vi "SDI-12 Multiple Operations.vi"() -> ()   [LabVIEW 2015]
doc: "A general set of examples of the SDI-12 API for a generic sensor. A tab control separates each example, and contains the following examples:\n1. Read Single.\n2. Read Multiple.\n3. Acknowledge Active.\n4. Change Address.\n5. Address Query.\n6. Send Identification."
uses:
  SDI-12.lvlib
panel:
  in  "Example Mode":T1(tab)=enum."Read Multiple"
  out "Address Out":string="a" caption="sensor address out"
  out "Number of Measurements Out":i32
  out "Measurements Out":dbl[](array[numeric])
  in  "Measurement Type In (Normal)":i32(ring) items=["Normal", "Concurrent", "Continuous"]
  out "Parameter Out":i32(ring) items=["0", "1", "2", "3", "4", "5", "6", "7", "8", "9"]
  in  "Parameter In (0)":i32(ring) items=["0", "1", "2", "3", "4", "5", "6", "7", "8", "9"]
  in  "CRC (False)":bool
  out "CRC Out":bool
  out "Measurement Type Out":i32(ring) items=["Normal", "Concurrent", "Continuous"]
  out "Time (s)":dbl
  out "Read Multiple: Error Array Out":errorcluster[](array[cluster])
  out "Number of Measurements Out Array":i32[](array[numeric])
  out "Measurements Out":dbl[][](array[numeric])
  in  "Measurement Type In (Normal)":i32(ring) items=["Normal", "Concurrent", "Continuous"]
  in  "Sensor Address In Array":string[](array[string])=["b", "b", "b"]
  in  "Parameter In Array (0)":i32[](array[ring])=[0, 0, 0] items=["0", "1", "2", "3", "4", "5", "6", "7", "8", "9"]
  in  "CRC In Array (False)":bool[](array[boolean])=[TRUE, FALSE, TRUE]
  out "Sensor Active?":bool
  out "Address Changed Successfully?":bool
  in  "New Address In":string="b"
  out "Query Address Returned":string
  out "Query Response?":bool
  out "Identification: Address":string
  out "SDI-12 Compatibility Number":dbl
  out "Company Name":string
  out "Sensor Model Number":string
  out "Sensor Version":string
  out "Serial Number":string
  in  "Error In (No Error)":errorcluster
  in  "Sensor Address In":string="0"
  in  "RS232 Port In":refnum<visa-resource-name>="COM11"
  out "Error Out":errorcluster
  # "Instructions:\n1.  Select the RS232 port that is connected to the SDI-12.\n2.  Enter a sensor address (not used for Read Multiple).\n3.  Select the desired test from the Example Mode Tab Control."
  # "4.  Select a Measurement type, a Parameter value,\n     and enable or disable CRC.\n5.  Run this VI."
  # "deg C"
  # "pH"
  # "specific conductance"
  # "salinity or TDS"
  # "DO % saturation"
  # "DO mg/L"
  # "ORP"
  # "depth"
  # "battery"
  # "4.  Enter an array of addresses of the sensors to measure.  All input arrays should be the same size.  The combined settings of each array at a single index value correspond to the settings of a single measurement. \n5.  Select a Measurement Type for all sensors.\n6.  Select an array of CRC settings.\n7.  Select an array of Parameter values if your sensor(s) support additional measurements by parameter value.  For example, for a single sensor parameter 0 (default) could be temperature, and parameter 1 could be humidity.\n8.  Run this VI."
  # "deg C"
  # "pH"
  # "specific conductance"
  # "salinity or TDS"
  # "DO % saturation"
  # "DO mg/L"
  # "ORP"
  # "depth"
  # "battery"
  # "4.  Run this VI."
  # "4.  Select the desired new address.\n5.  Run this VI."
  # "4.  Run this VI."
  # "4.  Run this VI."
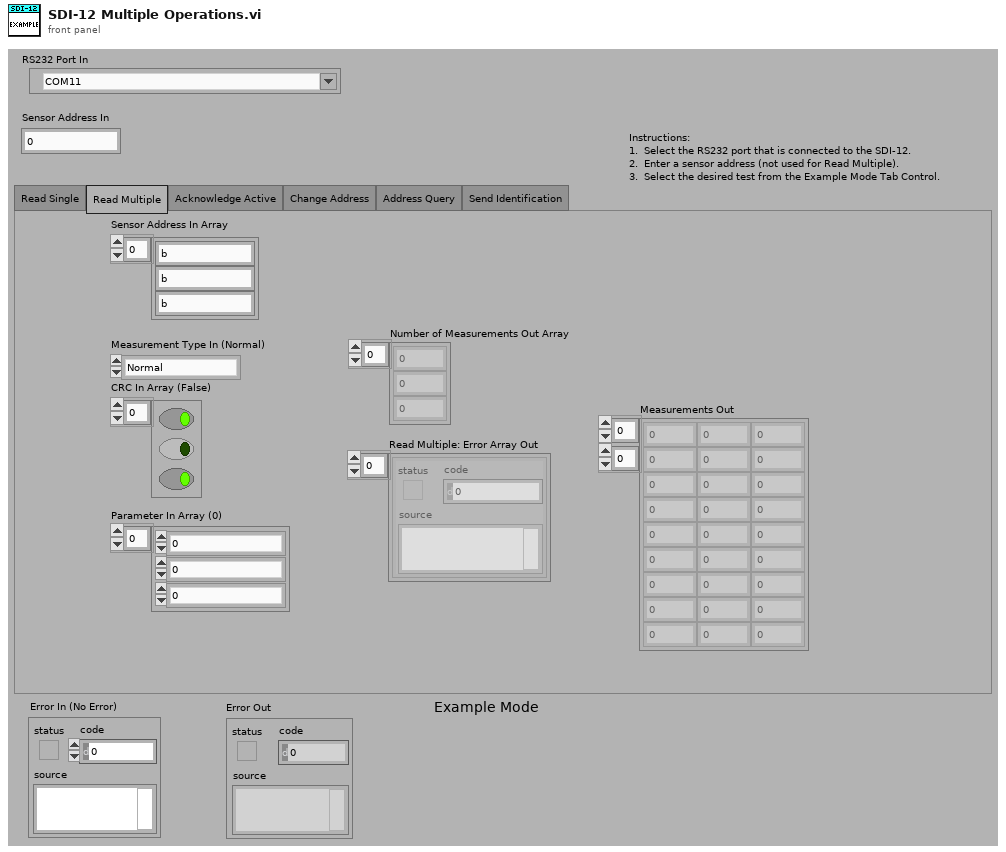
[diagram p1: front panel]
types:
  T1 = enum32{"Read Single", "Read Multiple", "Acknowledge Active", "Change Address", "Address Query", "Send Identification"}
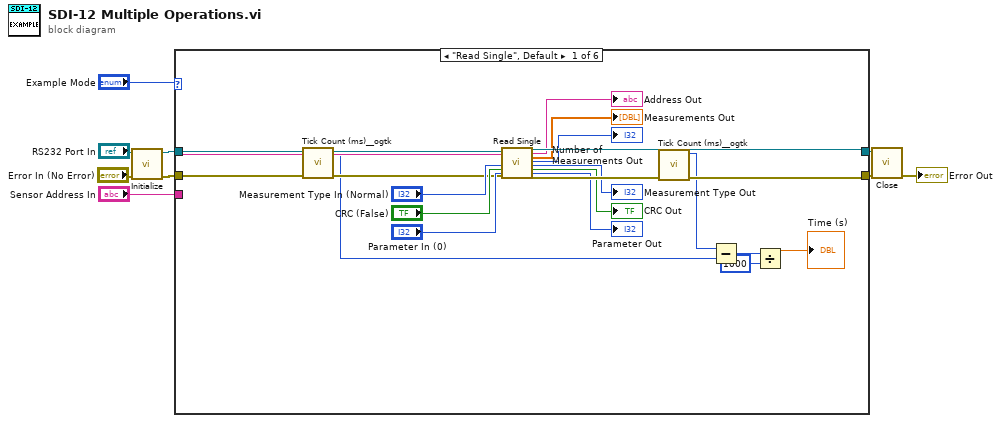
[diagram p0: block diagram]
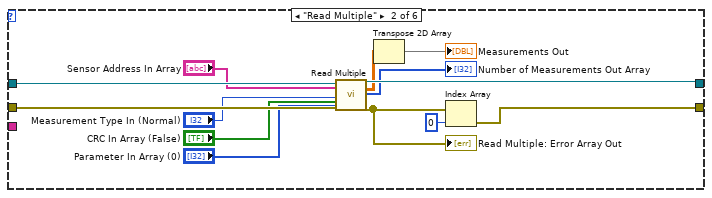
[diagram p2: hidden frame]
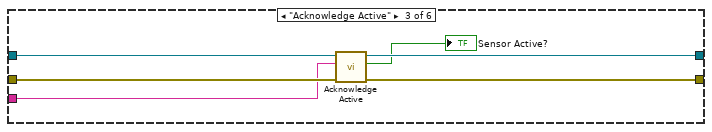
[diagram p3: hidden frame]
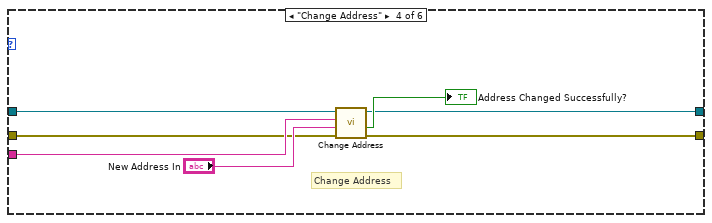
[diagram p4: hidden frame]
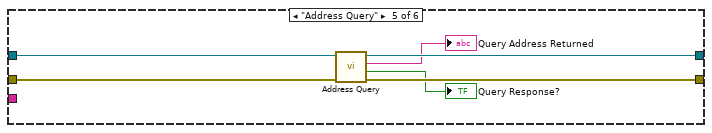
[diagram p5: hidden frame]
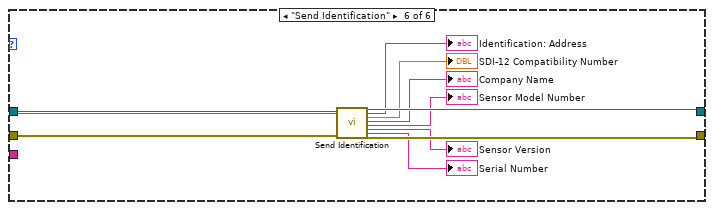
[diagram p6: hidden frame]
diagram:
  n1 = call "Initialize.vi"("Error In (No Error)"="Error In (No Error)", "RS232 Port In"="RS232 Port In") -> ("Error Out"=w3:errorcluster, "RS232 Port Out"=w4:refnum<visa-resource-name>)  [unwired: 8 in]
  n2 = case shown="\"Read Single\", Default" "Example Mode" {
    tunnel: "Sensor Address In" -> [w26 _ w44 w54 _ w63]
    tunnel: w4 -> [w30 w43 w49 w56 w62 w73]
    tunnel: w3 -> [w29 w42 w48 w52 w60 w71]
    tunnel: [w15 w39 w47 w51 w59 w70] -> w2
    tunnel: [w27 w38 w46 w50 w61 w72] -> w1
    frame "Read Single", Default {
      n3 = call <userlib>:"Tick Count (ms)__ogtk.vi"("error in (no error)"=w29) -> ("error out"=w16:errorcluster, "millisecond timer value"=w13:u32)  [unwired: 9 in]
      n4 = call "Read Single.vi"("RS232 Port In"=w30, "Sensor Address In"=w26, "Measurement Type In (Normal)"="Measurement Type In (Normal)", "CRC (False)"="CRC (False)", "Parameter In (0)"="Parameter In (0)", "Error In (No Error)"=w16) -> ("RS232 Port Out"=w27:refnum<visa-resource-name>, "Sensor Address Out"=→"Address Out":string, "Measurements Out"=→"Measurements Out":dbl[], "Number of Measurements Out"=→"Number of Measurements Out":i32, "Measurement Type Out"=→"Measurement Type Out":i32, "CRC Out"=→"CRC Out":bool, "Parameter Out"=→"Parameter Out":i32, "Error Out"=w28:errorcluster)  [unwired: 14 in]
      n5 = call <userlib>:"Tick Count (ms)__ogtk.vi"("error in (no error)"=w28) -> ("error out"=w15:errorcluster, "millisecond timer value"=w14:u32)  [unwired: 9 in]
      n6 = Subtract(x=w14, y=w13) -> (x-y=w12:u32)
      n7 = Divide(x=w12, y=u32 1000) -> (x/y=→"Time (s)":dbl)
    }
    frame "Read Multiple" {
      n8 = call "Read Multiple.vi"("RS232 Port In"=w43, "Sensor Address In Array"="Sensor Address In Array", "Measurement Type In (Normal)"="Measurement Type In (Normal)", "CRC In Array (False)"="CRC In Array (False)", "Parameter In Array (0)"="Parameter In Array (0)", "Error In (No Error)"=w42) -> ("RS232 Port Out"=w38:refnum<visa-resource-name>, "Measurements Out"=w33:dbl[][], "Number of Measurements Out Array"=→"Number of Measurements Out Array":i32[], "Error Out Array"=w41:errorcluster[])  [unwired: 14 in, 4 out]
      "Read Multiple: Error Array Out" <- w41
      n9 = Transpose 2D Array(2D array=w33) -> (transposed array=→"Measurements Out":dbl[][])
      n10 = Index Array(array=w41, index=0) -> (element=w39:errorcluster)
    }
    frame "Acknowledge Active" {
      n11 = call "Acknowledge Active.vi"("Error In (No Error)"=w48, "Sensor Address In"=w44, "RS232 Port In"=w49) -> ("Error Out"=w47:errorcluster, "Sensor Reply?"=→"Sensor Active?":bool, "RS232 Port Out"=w46:refnum<visa-resource-name>)  [unwired: 6 in]
    }
    frame "Change Address" {
      # "Change Address"
      n12 = call "Change Address.vi"("Error In (No Error)"=w52, "New Address In"="New Address In", "Sensor Address In"=w54, "RS232 Port In"=w56) -> ("Error Out"=w51:errorcluster, "Success?"=→"Address Changed Successfully?":bool, "RS232 Port Out"=w50:refnum<visa-resource-name>)  [unwired: 5 in]
    }
    frame "Address Query" {
      n13 = call "Address Query.vi"("Error In (No Error)"=w60, "RS232 Port In"=w62) -> ("Error Out"=w59:errorcluster, "Sensor Response?"=→"Query Response?":bool, "Sensor Address Out"=→"Query Address Returned":string, "RS232 Port Out"=w61:refnum<visa-resource-name>)  [unwired: 6 in]
    }
    frame "Send Identification" {
      n14 = call "Send Identification.vi"("RS232 Port In"=w73, "Sensor Address In"=w63, "Error In (No Error)"=w71) -> ("RS232 Port Out"=w72:refnum<visa-resource-name>, "Address Out"=→"Identification: Address":string, "SDI-12 Compatibility Number"=→"SDI-12 Compatibility Number":dbl, "Company Name"=→"Company Name":string, "Sensor Model Number"=→"Sensor Model Number":string, "Sensor Version"=→"Sensor Version":string, "Serial Number/MISC"=→"Serial Number":string, "Error Out"=w70:errorcluster)  [unwired: 17 in]
    }
  }
  n15 = call "Close.vi"("Error In (No Error)"=w2, "RS232 Port In"=w1) -> ("Error Out"=→"Error Out":errorcluster)  [unwired: 9 in]
